vi "poly_this_vis_name.vi"() -> (7 "your name":string)   [LabVIEW 2015]
doc: "Gives the name of the current vi. Be carefull when using this vi in inlined vi's as it will then give the name of the first not-inlined caller in the call chain.\n\nWritten by Marcin Konowalczyk\nTimmel Group @ Oxford University\n\nhttps://github.com/MarcinKonowalczyk/labview-utils"
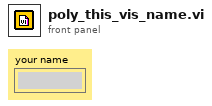
[diagram p1: front panel]
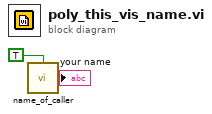
[diagram p0: block diagram]
diagram:
  n1 = call "name_of_caller.vi"("is in inlined vi? (F)"=TRUE) -> ("name of caller out"=→"your name":string)  [unwired: 3 in]
